vi "Lua class path.vi"() -> (3 "palette file path":path)   [LabVIEW 2020, in "Lua DevUtil.lvlib"]
uses:
  Lua DevUtil.lvlib
  Lua for LabVIEW/Lua/New Lua State.vi
  Lua for LabVIEW/Lua/Lua.lvclass
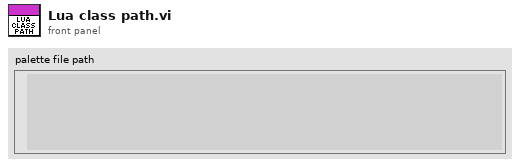
[diagram p1: front panel]
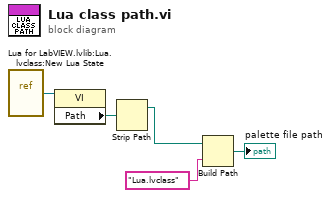
[diagram p0: block diagram]
diagram:
  n1 = vi-ref "Lua for LabVIEW.lvlib:Lua.lvclass:New Lua State.vi"() -> (w5:refnum<vi>)
  n2 = property class="VI"(reference=w5) -> ("Path"=w4:path)  [unwired: 1 in, 2 out]
  n3 = Strip Path(path=w4) -> (stripped path=w1:path)  [unwired: 1 out]
  n4 = Build Path(base path=w1, name or relative path="Lua.lvclass") -> (appended path=→"palette file path":path)
